vi "ROI Overlay.vi"(8 "error in (no error)":errorcluster, 10 "Master Bounds Rect":T2, 11 "ImageOperation in":refnum<class "ImageOperation.lvclass">) -> (0 "error out":errorcluster, 2 "ROI Descriptor":T1 {"Contours"."Type" items=["No Selection", "Point", "Line", "Rectangle", "Oval", "Polygon", "Freehand Region", "Annulus", "Unused2", "Unused3", "Broken Line", "Freehand Line", "Rotated Rectangle"]}, 3 "ImageOperation out":refnum<class "ImageOperation.lvclass">)   [LabVIEW 2015, in "ImageOperation.lvclass"]
uses:
  ImageOperation.lvclass
  <vilib>/Utility/miscctls.llb/LVRectTypeDef.ctl
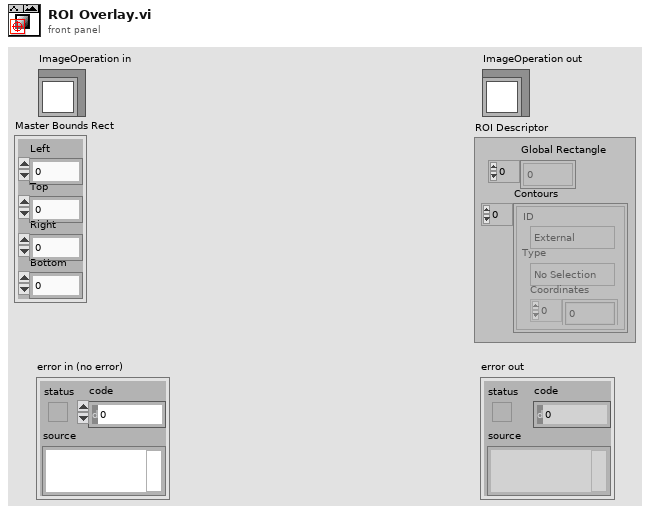
[diagram p1: front panel]
types:
  T1 = typedef "ROI Descriptor" = cluster{"Global Rectangle":i32[], "Contours":cluster{"ID":enum32{"External", "Internal"}, "Type":u32, "Coordinates":i32[]}[]}
  T2 = typedef "LVRectTypeDef.ctl" = cluster{"Left":i16, "Top":i16, "Right":i16, "Bottom":i16}
  T3 = typedef "IMAQ Rectangle" = cluster{"Left":i32, "Top":i32, "Right":i32, "Bottom":i32, "Rotation":dbl}
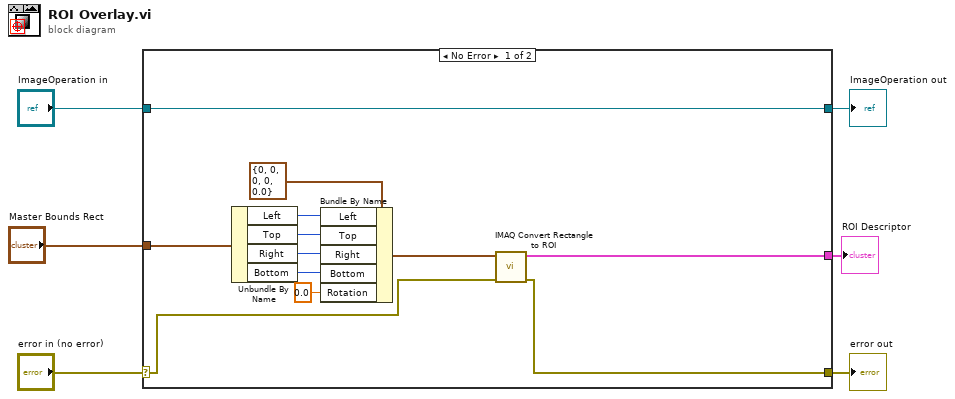
[diagram p0: block diagram]
diagram:
  n1 = case shown="No Error" "error in (no error)" {
    selector: "error in (no error)" -> [w16 w20]
    tunnel: [w8 w20] -> w5
    tunnel: [w18 w19] -> w3
    tunnel: "ImageOperation in" -> [w18 w19]
    tunnel: "Master Bounds Rect" -> [w17 _]
    tunnel: [w7 _] -> w1
    frame No Error {
      n2 = Unbundle By Name(w17) -> ("Left"=w14:i16, "Top"=w13:i16, "Right"=w12:i16, "Bottom"=w11:i16)
      n3 = Bundle By Name(cluster=T3 {"Left"=0, "Top"=0, "Right"=0, "Bottom"=0, "Rotation"=0.0} ("Rectangle"), "Left"=w14, "Top"=w13, "Right"=w12, "Bottom"=w11, "Rotation"=0.0) -> (w9:T3)
      n4 = call "IMAQ Convert Rectangle to ROI"("error in (no error)"=w16, "Rectangle"=w9) -> ("error out"=w8:errorcluster, "ROI Descriptor"=w7:T1)  [unwired: 7 in]
    }
    frame Error {
    }
  }
  "error out" <- w5
  "ImageOperation out" <- w3
  "ROI Descriptor" <- w1
